vi "Get Data.vi"(7 "LabVIEW Web Service Request":refnum<class "Web Request.lvclass">, 10 "Format":string caption="Format (use accept header)", 11 "Measurement":string caption="Measurement (all)") -> ()   [LabVIEW 2023]
doc: "HTTP method VI that retrieves all of the weather data and outputs it using stream mode. The output format is based on the value of an input terminal or, if the terminal is omitted, the Accept HTTP request header."
uses:
  <vilib>/wsapi/Web Request.lvclass
  Application/Weather Data.lvlib
  <vilib>/wsapi/NI_WebServices.lvlib
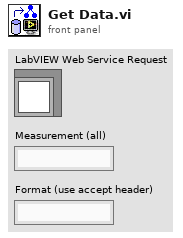
[diagram p1: front panel]
types:
  T1 = typedef "Weather Data.lvlib/Weather Data.ctl" = cluster{"Temperature":dbl, "Pressure":dbl, "Wind Speed":dbl, "Wind Direction":dbl}
  T2 = typedef "imagedata.ctl" = cluster{"image type":i32, "image depth":i32, "image":u8[], "mask":u8[], "colors":u32[], "Rectangle":cluster{"left":i16, "top":i16, "right":i16, "bottom":i16}}
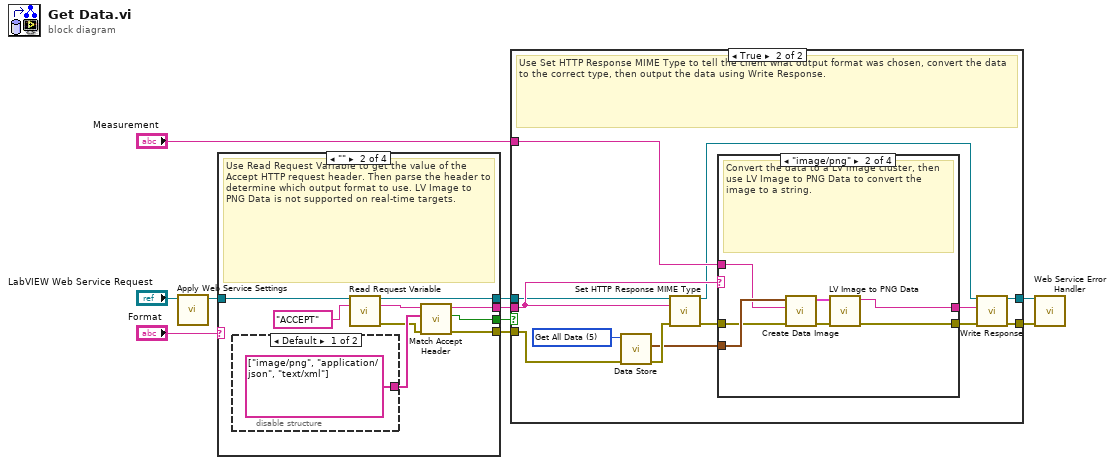
[diagram p0: block diagram]
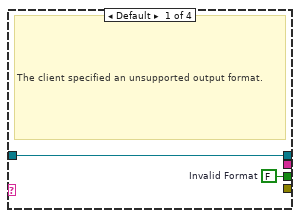
[diagram p2: hidden frame]
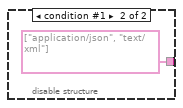
[diagram p3: hidden frame]
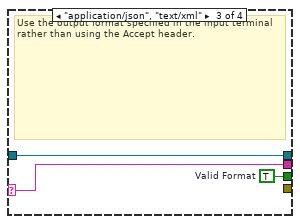
[diagram p4: hidden frame]
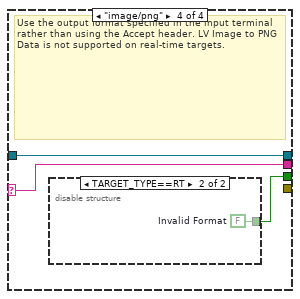
[diagram p5: hidden frame]
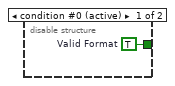
[diagram p6: hidden frame]
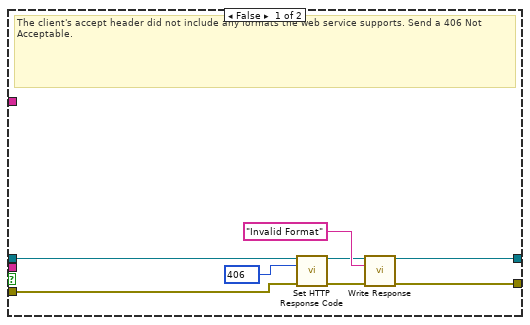
[diagram p7: hidden frame]
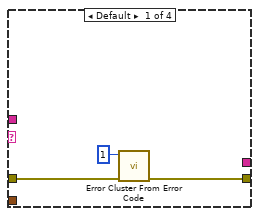
[diagram p8: hidden frame]
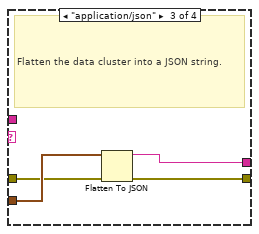
[diagram p9: hidden frame]
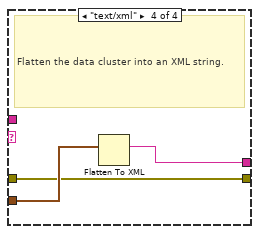
[diagram p10: hidden frame]
diagram:
  n1 = call "Apply Web Service Settings.vi"("LabVIEW Web Service Request"="LabVIEW Web Service Request") -> ("LabVIEW Web Service Request out"=w1:refnum<class "Web Request.lvclass">)  [unwired: 9 in, 1 out]
  n2 = case shown="\"\"" "Format" {
    selector: "Format" -> [_ _ w25 w28]
    tunnel: w1 -> [w12 w13 w26 w29]
    tunnel: [w11 w18 w24 w27] -> w9
    tunnel: [w12 w17 w26 w29] -> w8
    tunnel: [_ w15 _ _] -> w7
    tunnel: [_ w14 w25 w28] -> w6
    frame Default {
      w11 = FALSE  # Invalid Format
      # "The client specified an unsupported output format."
    }
    frame "" {
      # "Use Read Request Variable to get the value of the Accept HTTP request header. Then parse the header to determine which output format to use. LV Image to PNG Data is not supported on real-time targets."
      n3 = disable-structure shown="Default" {
        disable-tunnel: [string[] ["image/png", "application/json", "text/xml"] ("Valid Media Types") string[] ["application/json", "text/xml"] ("Valid Media Types")] -> w19
        frame condition #0 (active) {
        }
        frame condition #1 {
        }
      }
      n4 = call <vilib>:"Read Request Variable.vi"("LabVIEW Web Service Request"=w13, "variable name"="ACCEPT") -> ("LabVIEW Web Service Request out"=w17:refnum<class "Web Request.lvclass">, "value"=w20:string, "error out"=w16:errorcluster)  [unwired: 11 in]
      n5 = call "Match Accept Header.vi"("error in (no error)"=w16, "Valid Media Types"=w19, "Accept Value"=w20) -> ("error out"=w15:errorcluster, "Matched?"=w18:bool, "Matched Media Type"=w14:string)  [unwired: 6 in]
    }
    frame "application/json", "text/xml" {
      w24 = TRUE  # Valid Format
      # "Use the output format specified in the input terminal rather than using the Accept header."
    }
    frame "image/png" {
      # "Use the output format specified in the input terminal rather than using the Accept header. LV Image to PNG Data is not supported on real-time targets."
      n6 = disable-structure shown="TARGET_TYPE==RT" {
        disable-tunnel: [w30 w31] -> w27
        frame condition #0 (active) {
          w30 = TRUE  # Valid Format
        }
        frame condition #1 {
          w31 = FALSE  # Invalid Format
        }
      }
    }
  }
  n7 = case shown="True" w9 {
    tunnel: w8 -> [w33 w41]
    tunnel: w7 -> [w38 w49]
    tunnel: w6 -> [_ w51]
    tunnel: "Measurement" -> [_ w42]
    tunnel: [w35 w44] -> w4
    tunnel: [w34 w43] -> w3
    frame False {
      w39 = 406 items=["100"=100, "101"=101, "200"=200, "201"=201, "202"=202, "203"=203, "204"=204, "205"=205, "206"=206, "300"=300, "301"=301, "302"=302, "303"=303, "304"=304, "305"=305, "306"=306, "307"=307, "400"=400, "401"=401, "402"=402, "403"=403, "404"=404, "405"=405, "406"=406, "407"=407, "408"=408, "409"=409, "410"=410, "411"=411, "412"=412, "413"=413, "414"=414, "415"=415, "416"=416, "417"=417, "500"=500, "501"=501, "502"=502, "503"=503, "504"=504, "505"=505] ("response code (200)")
      # "The client's accept header did not include any formats the web service supports. Send a 406 Not Acceptable."
      n8 = call <vilib>:"Set HTTP Response Code.vi"("LabVIEW Web Service Request"=w33, "response code (200)"=w39, "error in (no error)"=w38) -> ("LabVIEW Web Service Request out"=w32:refnum<class "Web Request.lvclass">, "error out"=w37:errorcluster)  [unwired: 11 in]
      n9 = call <vilib>:"Write Response.vi"("LabVIEW Web Service Request"=w32, "response string"="Invalid Format", "error in (no error)"=w37) -> ("LabVIEW Web Service Request out"=w34:refnum<class "Web Request.lvclass">, "error out"=w35:errorcluster)  [unwired: 11 in]
    }
    frame True {
      w50 = u16 5 items=["Initialize Data Store", "Destroy Data Store", "Clear Data", "Append Data", "Get Last Data", "Get All Data"] ("action")
      # "Use Set HTTP Response MIME Type to tell the client what output format was chosen, convert the data to the correct type, then output the data using Write Response."
      n10 = call "Data Store.vi"("error in (no error)"=w49, "action"=w50) -> ("error out"=w48:errorcluster, "weather data out"=w47:T1[])  [unwired: 8 in]
      n11 = call <vilib>:"Set HTTP Response MIME Type.vi"("LabVIEW Web Service Request"=w41, "MIME type (text/html)"=w51, "error in (no error)"=w48) -> ("LabVIEW Web Service Request out"=w40:refnum<class "Web Request.lvclass">, "error out"=w52:errorcluster)  [unwired: 11 in]
      n12 = case shown="\"image/png\"" w51 {
        tunnel: w52 -> [w55 w57 w65 w68]
        tunnel: w47 -> [_ w60 w66 w69]
        tunnel: [w54 w58 w63 w68] -> w45
        tunnel: [_ w59 w64 w67] -> w46
        tunnel: w42 -> [_ w56 _ _]
        frame Default {
          n13 = call <vilib>:"Error Cluster From Error Code.vi"("error in (no error)"=w55, "error code (0)"=1) -> ("error out"=w54:errorcluster)  [unwired: 7 in]
        }
        frame "image/png" {
          # "Convert the data to a LV image cluster, then use LV Image to PNG Data to convert the image to a string."
          n14 = call "Create Data Image.vi"("error in (no error)"=w57, "Measurement"=w56, "Weather Data"=w60) -> ("error out"=w62:errorcluster, "image data"=w61:T2)  [unwired: 7 in]
          n15 = call <vilib>:"LV Image to PNG Data.vi"("error in (no error)"=w62, "image data"=w61) -> ("error out"=w58:errorcluster, "png data"=w59:string)  [unwired: 8 in]
        }
        frame "application/json" {
          # "Flatten the data cluster into a JSON string."
          n16 = Flatten To JSON(anything=w66, error in (no error)=w65) -> (JSON string=w64:string, 11:w63:errorcluster)  [unwired: 1 in]
        }
        frame "text/xml" {
          # "Flatten the data cluster into an XML string."
          n17 = Flatten To XML(6:w69) -> (2:w67:string)
        }
      }
      n18 = call <vilib>:"Write Response.vi"("LabVIEW Web Service Request"=w40, "response string"=w46, "error in (no error)"=w45) -> ("LabVIEW Web Service Request out"=w43:refnum<class "Web Request.lvclass">, "error out"=w44:errorcluster)  [unwired: 11 in]
    }
  }
  n19 = call "Web Service Error Handler.vi"("LabVIEW Web Service Request"=w3, "error in (no error)"=w4) -> ()  [unwired: 12 in, 2 out]
